vi "Banda Transportadora.vi"() -> ()   [LabVIEW 2019]
panel:
  in  "stop":bool
  out "Tope Derecho":bool
  out "Tope Izquierdo":bool
  in  "Velocidad (m/300ms)":dbl(knob) scale=0.0..10.0 scale format="%#_2g"
  in  "Dirección":bool
  in  "Acción":bool
  in  "Banda Transportadora":dbl(slide) scale=0.0..1200.0
  # "Continuar"
  # "Derecha"
  # "Detener"
  # "Izquierda"
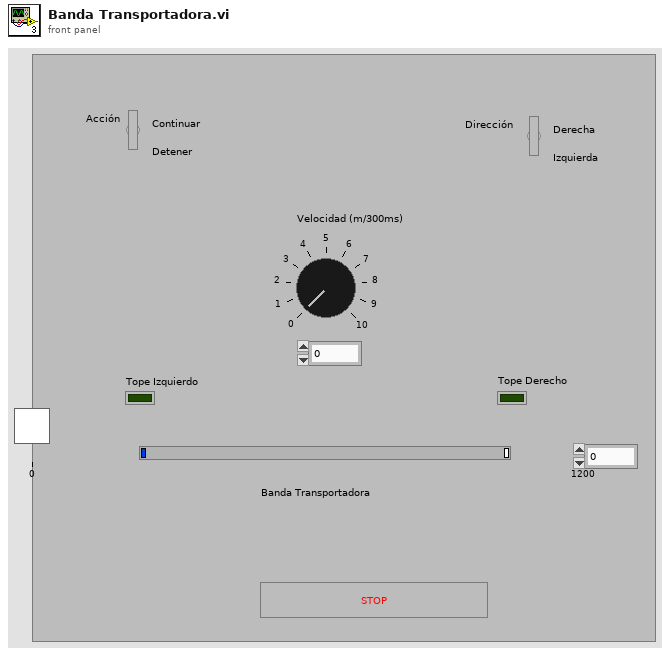
[diagram p1: front panel]
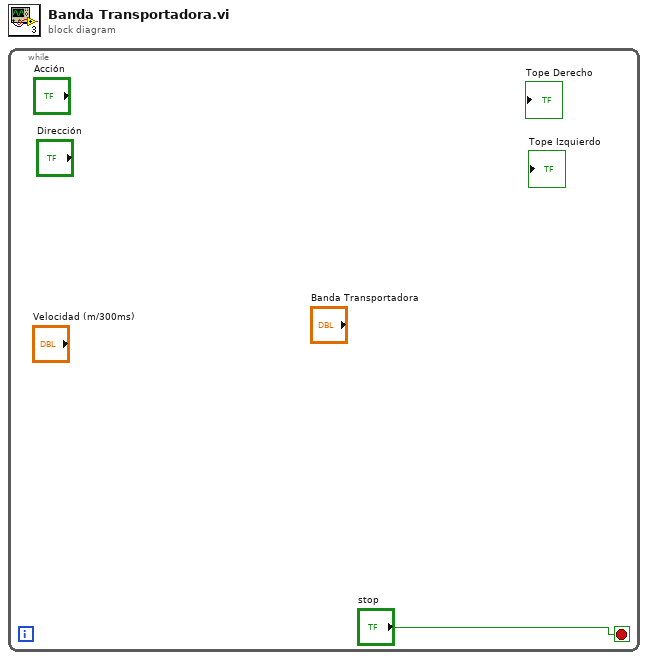
[diagram p0: block diagram]
diagram:
  n1 = while {
    stop <- "stop" stop-if-true
  }
